vi "Close.vi"(8 "error in (no error)":errorcluster, 11 "Route Manager in":refnum<class "Route Manager.lvclass">) -> (0 "error out":errorcluster)   [LabVIEW 2015, in "Route Manager.lvclass"]
uses:
  Route Manager.lvclass
  Route Manager.lvclass/Route Manager.ctl
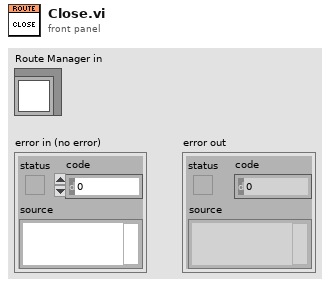
[diagram p1: front panel]
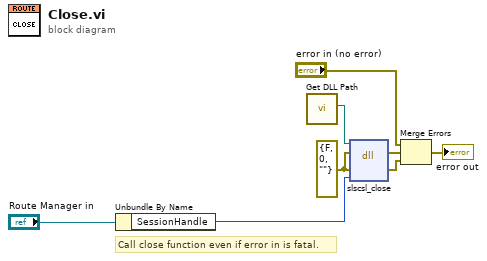
[diagram p0: block diagram]
diagram:
  w1 = errorcluster {"status"=FALSE, "code"=0, "source"=""} ("error in (no error)")
  # "Call close function even if error in is fatal."
  n1 = Unbundle By Name("Route Manager in") -> ("SessionHandle"=w2:u64)
  n2 = call "Get DLL Path.vi"() -> ("slscsl DLL Path"=w3:path)  [unwired: 11 in]
  n3 = dll-call lib="?" fn="slscsl_close"(path in=w3, error in=w1, "errorCluster"=w1, "sessionHandle"=w2) -> (error out=w5:errorcluster, "errorCluster"=w4:errorcluster)  [unwired: 3 in, 1 out]
  n4 = Merge Errors("error in (no error)", w5, w4) -> (→"error out":errorcluster)
